vi "Init.vi"(0 "Session In":refnum<class "SmartScopeDriver.lvclass">, 11 "error in (no error)":errorcluster) -> (4 "Session Out":refnum<class "SmartScopeDriver.lvclass">, 15 "error out":errorcluster)   [LabVIEW 2019, in "SmartScopeDriver.lvclass"]
doc: "Initializes the Smart Scope."
uses:
  SmartScopeDriver.lvclass
  SmartScopeDriver.lvclass/SmartScopeDriver.ctl
  Scope Driver/LabNation Scope Driver.lvlib
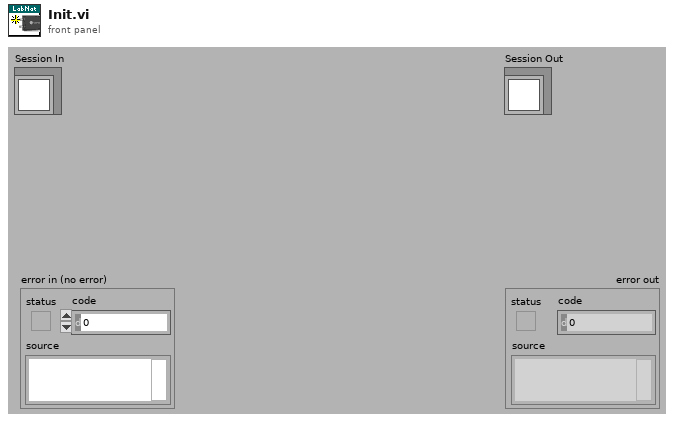
[diagram p1: front panel]
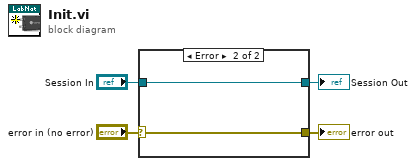
[diagram p0: block diagram]
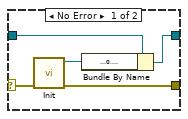
[diagram p2: hidden frame]
diagram:
  n1 = case shown="Error" "error in (no error)" {
    selector: "error in (no error)" -> [w5 w11]
    tunnel: "Session In" -> [w9 w10]
    tunnel: [w6 w11] -> w4
    tunnel: [w8 w10] -> w2
    frame No Error {
      n2 = call "Init.vi"("error in (no error)"=w5) -> ("error out"=w6:errorcluster, "reference out"=w7:refnum<k24>)  [unwired: 9 in]
      n3 = Bundle By Name(cluster=w9, "reference"=w7) -> (w8:refnum<class "SmartScopeDriver.lvclass">)
    }
    frame Error {
    }
  }
  "error out" <- w4
  "Session Out" <- w2
